vi "W vs Z main4f.vi"() -> ()   [LabVIEW 2016]
panel:
  out "Contains waist?":bool[](array[boolean])
  out "FWHM":dbl[](array[numeric])
  out "min w":dbl[](array[numeric])
  out "min z":dbl[](array[numeric])
  out "w Matrix":dbl[][](array[numeric])
  out "Z Matrix":dbl[][](array[numeric])
  out "Number of lenses":i32
  in  "Lens Focal lengths":dbl[](array[numeric]) format="%.3f"
  in  "FWHM(T)?":bool
  out "Cursor List":T1(array[cluster]) {"Location"."Y" format="%.2f"; "Location"."X" format="%.2f"}
  in  "z stop":dbl=1000.0 format="%.2f"
  in  "N steps":i32=500
  out "Q start":cdb format="%.4f"
  out "W vs Z":cluster{dbl[], dbl[]}[](graph)
  in  "beam radius(w)":dbl=0.6 format="%.5f"
  in  "Radius of Curvature":dbl=inf format="%.2f"
  in  "Wavelength":dbl=0.00035 format="%.6f"
  in  "z start":dbl format="%.2f"
  # "All values are entered in mm"
  # "w is the 1/e field radius"
  # "w x 1.18 to get FWHM of the Intensity"
  # "Zs plotted above. Each row is a segment between adjacent lenses"
  # "Ws plotted above. Each row is a segment between adjacent lenses"
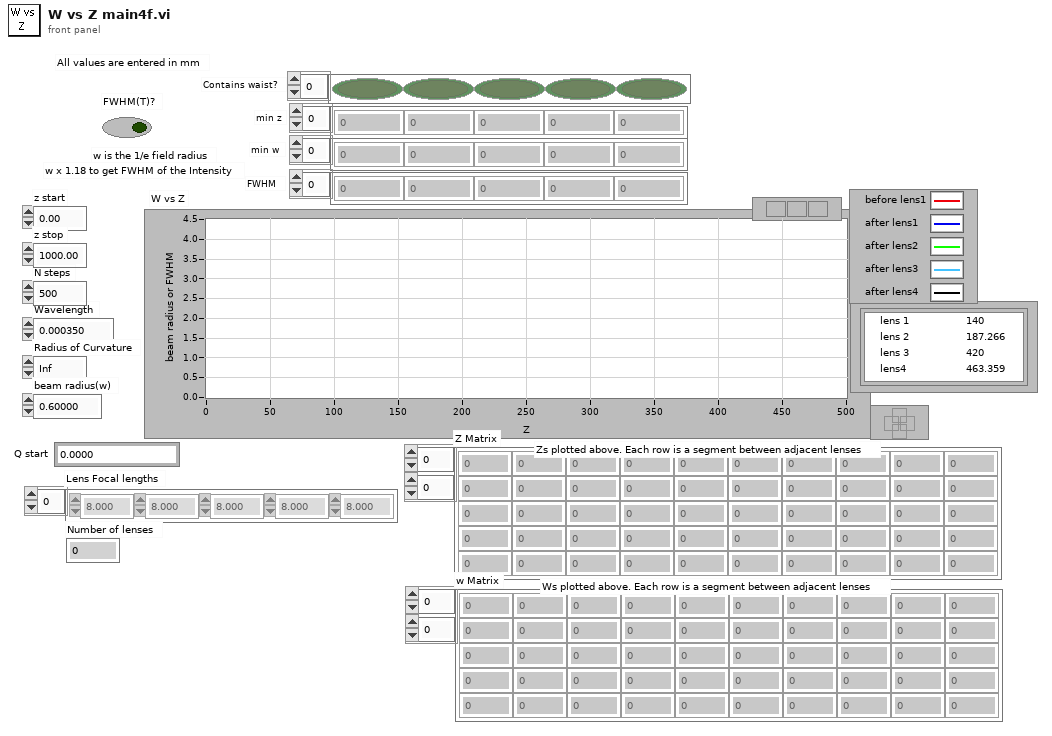
[diagram p1: front panel]
types:
  T1 = cluster{"Name":string, "Color":u32, "Hair Style":u8, "Point Style":u8, "Name Visible":bool, "Trackable":bool, "Lock Style":u32, "Plot Number":u32, "Marker Index":i32, "Location":cluster{"X":dbl, "Y":dbl}}[]
  T2 = cluster{"Name":string, "Color":u32, "Style":u8, "Point Style":u8, "Name Visible":bool, "Allow Drag":bool, "Lock Style":u32, "Plot":u32, "Index":i32, "Position":cluster{"X":dbl, "Y":dbl}}[]
  T3 = cluster{"Name":string, "Color":u32, "Style":u8, "Point Style":u8, "Name Visible":bool, "Allow Drag":bool, "Lock Style":u32, "Plot":u32, "Index":i32, "Position":cluster{"X":dbl, "Y":dbl}}
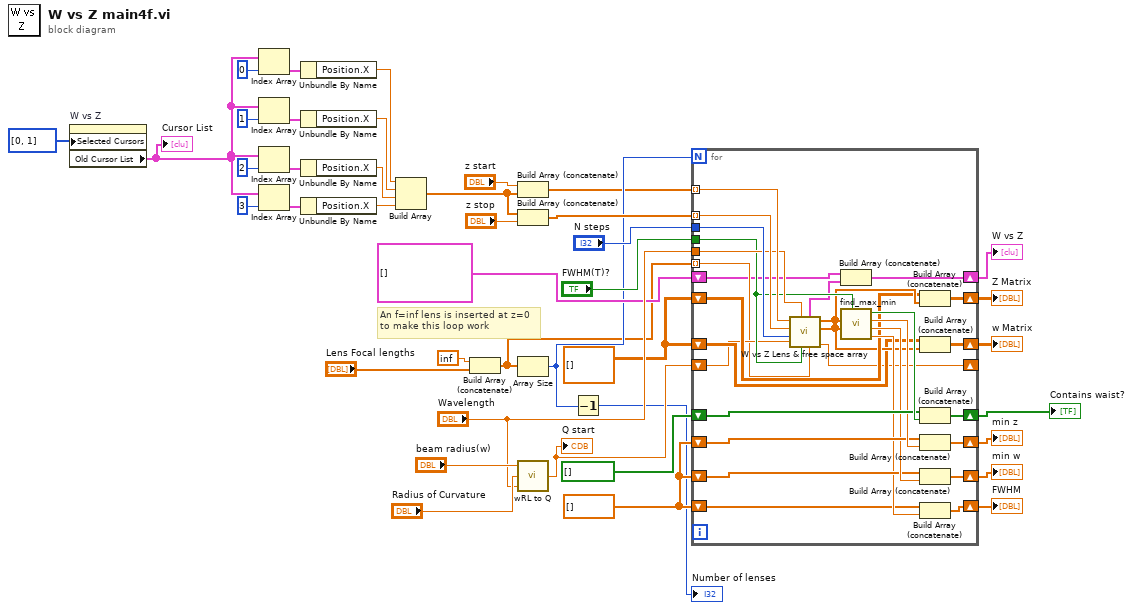
[diagram p0: block diagram]
diagram:
  w8 = dbl[] []
  w7 = dbl[][] []
  # "An f=inf lens is inserted at z=0\nto make this loop work"
  n1 = property on="W vs Z" class="XYGraph (strict)"("Selected Cursors"=u32[] [0, 1]) -> ("Old Cursor List"=w29:T2)  [unwired: 2 in, 2 out]
  "Cursor List" <- w29
  n2 = Index Array(array=w29, index=0 ("Index")) -> (element=w38:T3)
  n3 = Index Array(array=w29, index=1 ("Index")) -> (element=w36:T3)
  n4 = Index Array(array=w29, index=2 ("Index")) -> (element=w32:T3)
  n5 = Index Array(array=w29, index=3 ("Index")) -> (element=w30:T3)
  n6 = Unbundle By Name(w38) -> ("Position.X"=w10:dbl)
  n7 = Unbundle By Name(w36) -> ("Position.X"=w24:dbl)
  n8 = Unbundle By Name(w32) -> ("Position.X"=w22:dbl)
  n9 = Unbundle By Name(w30) -> ("Position.X"=w21:dbl)
  n10 = Build Array(w10, w24, w22, w21) -> (w1:dbl[])
  n11 = Build Array (concatenate)(inf, "Lens Focal lengths") -> (w11:dbl[])
  n12 = Build Array (concatenate)("z start", w1) -> (w2:dbl[])
  n13 = Build Array (concatenate)(w1, "z stop") -> (w23:dbl[])
  n14 = Array Size(array=w11) -> (size(s)=w14:i32)
  n15 = call "wRL to Q.vi"("Wavelength"="Wavelength", "Radius of Curvature"="Radius of Curvature", "beam radius(w)"="beam radius(w)") -> ("Q"=w9:cdb)
  "Q start" <- w9
  n16 = Decrement(x=w14) -> (x-1=→"Number of lenses":i32)
  n17 = for {
    N: w14 -> [_]
    tunnel: "N steps" -> [w70]
    tunnel: w23 -> [w69] mode=indexing
    tunnel: w2 -> [w68] mode=indexing
    tunnel: "Wavelength" -> [w67]
    tunnel: "FWHM(T)?" -> [w66]
    shift-right: [w65] -> w4
    shift-left: bool[] [] -> [w63]
    shift-right: [w61] -> w18
    shift-left: w8 -> [w60]
    shift-right: [w58] -> w17
    shift-left: w8 -> [w57]
    shift-right: [w45] -> w16
    shift-left: w8 -> [w55]
    shift-right: [w53] -> w25
    shift-left: w7 -> [w52]
    shift-right: [w50] -> w19
    shift-left: w7 -> [w49]
    shift-right: [w48] -> _
    shift-left: w9 -> [w47]
    tunnel: w11 -> [w46] mode=indexing
    shift-right: [w43] -> w26
    shift-left: cluster{dbl[], dbl[]}[] [] -> [w42]
    n18 = call "W vs Z Lens & free space array.vi"("lens focal length"=w46, "FWHM(T)?"=w66, "Wavelength"=w67, "Q in"=w47, "N steps"=w70, "z stop"=w69, "z start"=w68) -> ("Q out"=w48:cdb, "w/FWHM Array"=w51:dbl[], "Z Array"=w54:dbl[], "W/FWHM vs Z"=w44:cluster{dbl[], dbl[]})  [unwired: 1 out]
    n19 = Build Array (concatenate)(w42, w44) -> (w43:cluster{dbl[], dbl[]}[])
    n20 = call "find_max_min.vi"("FWHM(T)?"=w66, "w Array"=w51, "z Array"=w54) -> ("FWHM"=w56:dbl, "min w"=w59:dbl, "min  z"=w62:dbl, "contains waist?"=w64:bool)  [unwired: 5 in]
    n21 = Build Array (concatenate)(w52, w54) -> (w53:dbl[][])
    n22 = Build Array (concatenate)(w49, w51) -> (w50:dbl[][])
    n23 = Build Array (concatenate)(w63, w64) -> (w65:bool[])
    n24 = Build Array (concatenate)(w60, w62) -> (w61:dbl[])
    n25 = Build Array (concatenate)(w57, w59) -> (w58:dbl[])
    n26 = Build Array (concatenate)(w55, w56) -> (w45:dbl[])
  }
  "W vs Z" <- w26
  "Z Matrix" <- w25
  "w Matrix" <- w19
  "min z" <- w18
  "min w" <- w17
  "FWHM" <- w16
  "Contains waist?" <- w4
